vi "User_Check.vi"(8 "error in (no error)":errorcluster, 9 "Array":string[][](array[string]), 10 "User_id":i32, 11 "User found":bool) -> (0 "error out":errorcluster, 2 "Cash":dbl, 3 "ATM window":string)   [LabVIEW 2025]
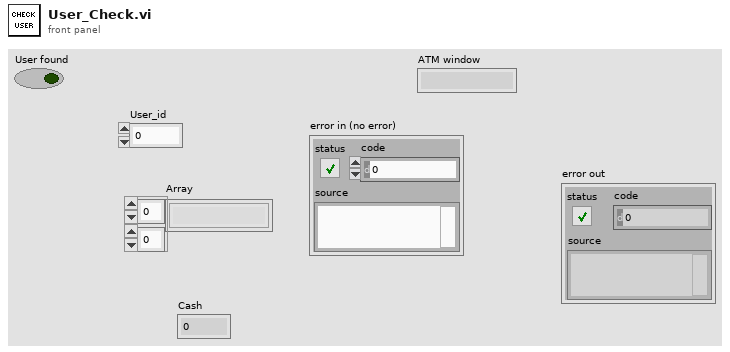
[diagram p1: front panel]
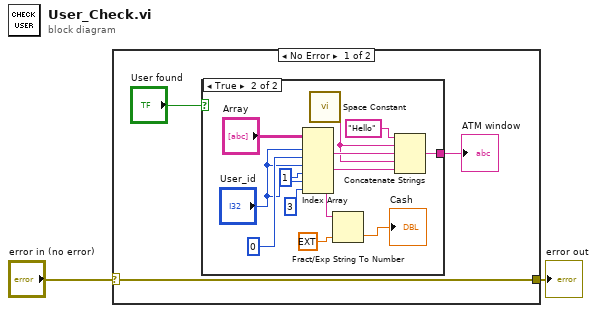
[diagram p0: block diagram]
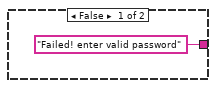
[diagram p2: hidden frame]
diagram:
  n1 = case shown="No Error" "error in (no error)" {
    selector: "error in (no error)" -> [w3 w20]
    tunnel: [w3 w20] -> w1
    frame No Error {
      n2 = case shown="True" "User found" {
        tunnel: ["Failed! enter valid password" ("element") w12] -> w4
        frame False {
        }
        frame True {
          n3 = Index Array(array="Array", index (row) #1="User_id", index (col) #1=0 ("index (col)"), index (row) #2="User_id", index (col) #2=1 ("index (col)"), index (row) #3="User_id", index (col) #3=3 ("index (col)")) -> (element #1=w15:string, element #2=w13:string, element #3=w9:string)
          n4 = call <vilib>:"Space Constant.vi"() -> ("String"=w14:string)
          n5 = Fract/Exp String To Number(string=w9, default (0 dbl)=ext 0.0 ("default (0 DBL)")) -> (number=→"Cash":ext)  [unwired: 2 in, 1 out]
          n6 = Concatenate Strings("Hello" ("element"), w14, w15, w14, w13) -> (w12:string)
        }
      }
      "ATM window" <- w4
    }
    frame Error {
    }
  }
  "error out" <- w1
